vi "Demo.vi"() -> ()   [LabVIEW 2010]
uses:
  My Algorithm Library/builds/My Algorithm Library.lvlibp
panel:
  in  "Knob":u32(knob) scale=0.0..100.0
  out "n!":ext format="%#.0f"
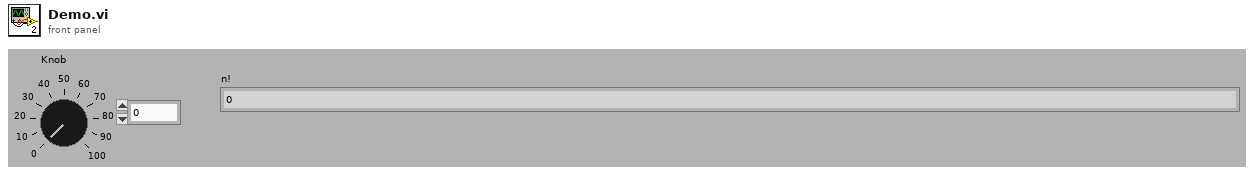
[diagram p1: front panel]
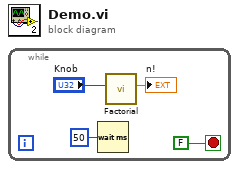
[diagram p0: block diagram]
diagram:
  n1 = while {
    stop <- FALSE stop-if-true
    n2 = Wait (ms)(milliseconds to wait=u32 50) -> ()  [unwired: 1 out]
    n3 = call "Factorial.vi"("n"="Knob") -> ("n!"=→"n!":ext)  [unwired: 10 in]
  }
